vi "ModuleCode.vi"(11 "ArgparseWrapper in":refnum<class "ArgparseWrapper.lvclass">) -> (2 "ModuleCode":string, 3 "ArgparseWrapper out":refnum<class "ArgparseWrapper.lvclass">)   [LabVIEW 2022 SP3, in "ArgumentParser.lvlib" / "ArgparseWrapper.lvclass"]
uses:
  ArgparseWrapper.lvclass
  ArgparseWrapper.lvclass/ArgparseWrapper.ctl
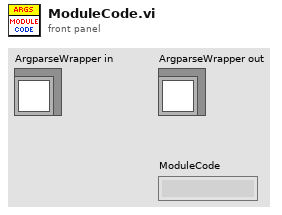
[diagram p1: front panel]
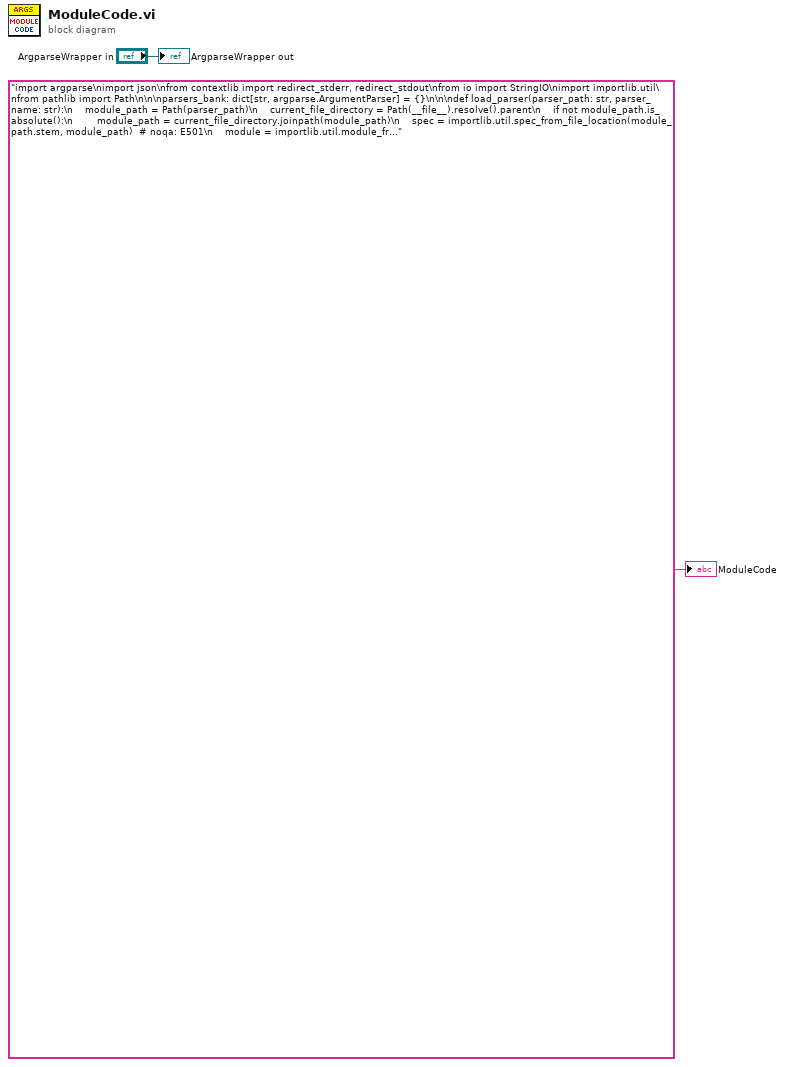
[diagram p0: block diagram]
diagram:
  "ArgparseWrapper out" <- "ArgparseWrapper in"
  "ModuleCode" <- "import argparse\nimport json\nfrom contextlib import redirect_stderr, redirect_stdout\nfrom io import StringIO\nimport importlib.util\nfrom pathlib import Path\n\n\nparsers_bank: dict[str, argparse.ArgumentParser] = {}\n\n\ndef load_parser(parser_path: str, parser_name: str):\n    module_path = Path(parser_path)\n    current_file_directory = Path(__file__).resolve().parent\n    if not module_path.is_absolute():\n        module_path = current_file_directory.joinpath(module_path)\n    spec = importlib.util.spec_from_file_location(module_path.stem, module_path)  # noqa: E501\n    module = importlib.util.module_from_spec(spec)\n    spec.loader.exec_module(module)\n    func = getattr(module, 'parser')\n    parsers_bank.update({parser_name: func()})\n\n\ndef parse_args(\n        parser_name: str,\n        arguments: list[str]\n        ):\n    err = out = parsed = ''\n    with (\n            redirect_stderr(StringIO()) as tmp_stderr,\n            redirect_stdout(StringIO()) as tmp_stdout\n            ):\n        try:\n            global parsers_bank\n            parsed = parsers_bank.get(parser_name).parse_args(arguments)\n            if parsed is not None:\n                parsed = json.dumps(vars(parsed))\n            else:\n                parsed = ''\n        except SystemExit as se:\n            if se.code == 0 or 2:\n                err = tmp_stderr.getvalue()\n                out = tmp_stdout.getvalue()\n            else:\n                raise se\n    return [parsed, out, err]\n\n\nif __name__ == '__main__':\n    out = err = parsed = ''\n\n    load_parser('parsers/example_parser.py', 'example_parser')\n    parsed = parse_args('example_parser', 'echo -h'.split())\n\n    out = parsed[1]\n    err = parsed[2]\n    parsed = parsed[0]\n\n    print(36*'#' + ' stdout ' + 36*'#')\n    print(out)\n    print(36*'#' + ' stderr ' + 36*'#')\n    print(err)\n    print(36*'#' + ' parsed ' + 36*'#')\n    print(parsed)\n" ("PythonCode")
